vi "Locate Named Attribute.vi"(10 "attribute name":string, 11 "error":errorcluster) -> (0 "found":bool, 1 "attribute tokens":cluster{"token type":T1, T2}[](array[cluster]), 2 "JSON Object Descriptor":T4={"begin info"={"match string"="", "raw token type"=enum."invalid", "byte offset "=0}, "end info"={"match string"="", "raw token type"=enum."invalid", "byte offset "=0}, "begin Index"=0, "end Index"=0}, 4 "attr index":i32, 5 "attributes":i32)   [LabVIEW 2020, in "Multi Error Cluster.lvlib"]
doc: "Return the value of the named attribute stored in the error cluster. If the named attribute isn't found, an empty string will be returned."
uses:
  <vilib>/MultiError/TokenizeJSON/Multi Error Cluster.lvlib
  <vilib>/MultiError/Errors Cluster Multiple Errors/JSON Object Descriptor.ctl
  <vilib>/MultiError/Errors Cluster Multiple Errors/JSON Token Descriptor.ctl
  <vilib>/MultiError/TokenizeJSON/JSON Raw Token Values.ctl
  <vilib>/MultiError/TokenizeJSON/JSON Token Values.ctl
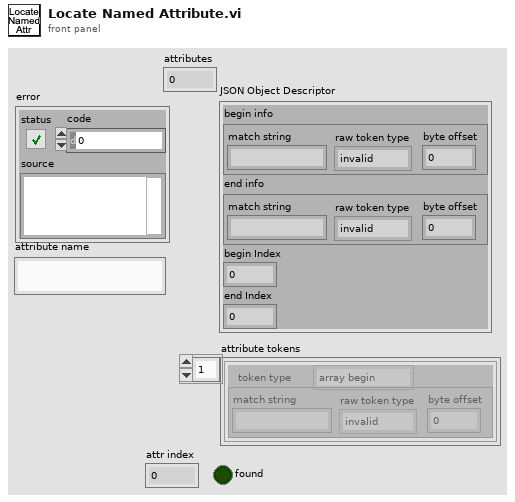
[diagram p1: front panel]
types:
  T1 = typedef "Multi Error Cluster.lvlib/JSON Token Values.ctl" = enum32{"array begin", "array end", "object begin", "object end", "value", "invalid", "name"}
  T2 = typedef "Multi Error Cluster.lvlib/JSON Token Descriptor.ctl" = cluster{"match string":string, "raw token type":T3, "byte offset ":i32}
  T3 = typedef "Multi Error Cluster.lvlib/JSON Raw Token Values.ctl" = enum32{"{", "}", "[", "]", ",", ":", "\"", "number", "string", "true", "false", "null", "invalid"}
  T4 = typedef "Multi Error Cluster.lvlib/JSON Object Descriptor.ctl" = cluster{"begin info":T2, "end info":T2, "begin Index":i32, "end Index":i32}
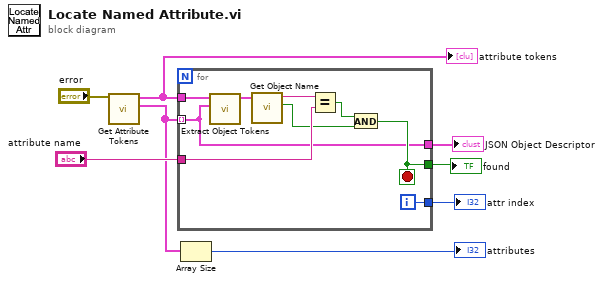
[diagram p0: block diagram]
diagram:
  n1 = call <vilib>:"Get Attribute Tokens.vi"("error"="error") -> ("array of JSON objects"=w2:T4[], "attribute tokens"=w8:cluster{"token type":T1, T2}[])  [unwired: 8 in, 1 out]
  "attribute tokens" <- w8
  n2 = for {
    tunnel: w8 -> [w12]
    tunnel: [w11] -> w7
    tunnel: w2 -> [w10] mode=indexing
    tunnel: "attribute name" -> [w15]
    tunnel: [w10] -> w4
    tunnel: [w9] -> w3
    i -> [w9]
    stop <- w11 stop-if-true
    n3 = call <vilib>:"Extract Object Tokens.vi"("JSON Object Descriptor"=w10, "attribute tokens"=w12) -> ("Extracted Tokens"=w17:cluster{"token type":T1, T2}[])  [unwired: 9 in]
    n4 = call <vilib>:"Get Object Name.vi"("Extracted Tokens"=w17) -> ("found"=w13:bool, "name"=w16:string)  [unwired: 9 in]
    n5 = Equal?(x=w16, y=w15) -> (x = y?=w14:bool)
    n6 = And(x=w14, y=w13) -> (x .and. y?=w11:bool)
  }
  "found" <- w7
  "JSON Object Descriptor" <- w4
  "attr index" <- w3
  n7 = Array Size(array=w2) -> (size(s)=→"attributes":i32)
